vi "raw_to_calibrated-scalar.vi"(5 "tag_name":string, 7 "runtime":variant, 8 "error in (no error)":errorcluster, 11 "value in":dbl) -> (0 "error out":errorcluster, 3 "value out":dbl)   [LabVIEW 2015, in "lv-calibration.lvlib"]
uses:
  lv-calibration.lvlib
  _controls/error.ctl
  <vilib>/gmath/NI_Gmath.lvlib
  <vilib>/Analysis/NI_AALPro.lvlib
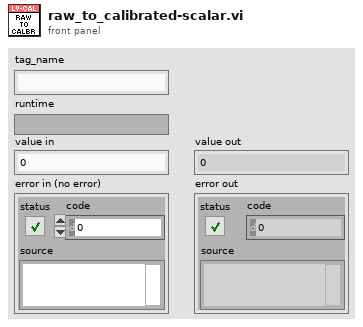
[diagram p1: front panel]
types:
  T1 = typedef "lv-calibration.lvlib/error.ctl" = enum16{"<error>", "unsupported_calibration_type", "tag_name_not_found", "duplicate_tag_names", "formula_empty"}
  T2 = typedef "lv-calibration.lvlib/runtime.ctl" = cluster{"tag_name":string, "type":T3, "offset":dbl, "slope":dbl, "formula":string, "x_points":dbl[], "y_points":dbl[]}
  T3 = typedef "lv-calibration.lvlib/type.ctl" = string
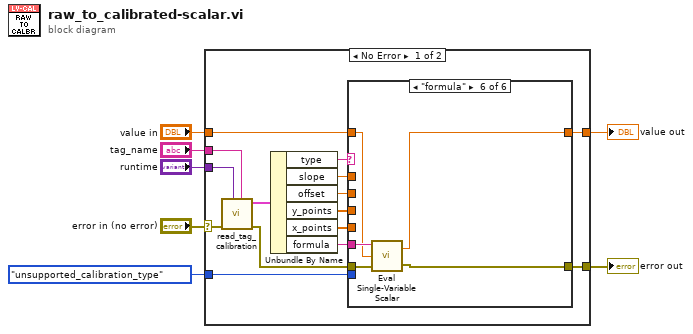
[diagram p0: block diagram]
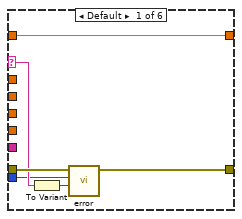
[diagram p2: hidden frame]
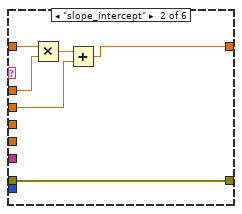
[diagram p3: hidden frame]
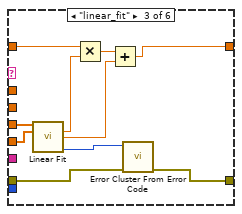
[diagram p4: hidden frame]
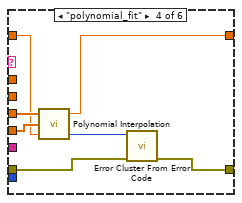
[diagram p5: hidden frame]
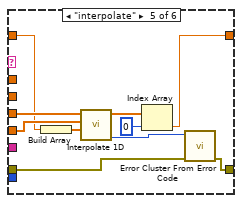
[diagram p6: hidden frame]
diagram:
  n1 = case shown="No Error" "error in (no error)" {
    selector: "error in (no error)" -> [w12 w67]
    tunnel: "value in" -> [w19 _]
    tunnel: [w18 _] -> w6
    tunnel: [w17 w67] -> w5
    tunnel: error."unsupported_calibration_type" ("error") -> [w16 _]
    tunnel: "runtime" -> [w14 _]
    tunnel: "tag_name" -> [w13 _]
    frame No Error {
      n2 = call "read_tag_calibration.vi"("tag_name"=w13, "runtime"=w14, "error in (no error)"=w12) -> ("error out"=w11:errorcluster, "calibration"=w15:T2)  [unwired: 7 in]
      n3 = Unbundle By Name(w15) -> ("type"=w22:T3, "slope"=w21:dbl, "offset"=w20:dbl, "y_points"=w10:dbl[], "x_points"=w9:dbl[], "formula"=w8:string)
      n4 = case shown="\"formula\"" w22 {
        selector: w22 -> [w26 _ _ _ _ _]
        tunnel: w11 -> [w27 w29 w36 w46 w53 w63]
        tunnel: w21 -> [_ w33 _ _ _ _]
        tunnel: w20 -> [_ w32 _ _ _ _]
        tunnel: w19 -> [w28 w34 w40 w49 w59 w65]
        tunnel: [w28 w30 w38 w48 w56 w64] -> w18
        tunnel: [w23 w29 w35 w45 w52 w62] -> w17
        tunnel: w16 -> [w24 _ _ _ _ _]
        tunnel: w10 -> [_ _ w44 w51 w61 _]
        tunnel: w9 -> [_ _ w43 w50 w60 _]
        tunnel: w8 -> [_ _ _ _ _ w66]
        frame Default {
          n5 = To Variant(anything=w26) -> (Variant=w25:variant)
          n6 = call "error.vi"("data"=w25, "error"=w24, "error in (no error)"=w27) -> ("error out"=w23:errorcluster)  [unwired: 8 in]
        }
        frame "slope_intercept" {
          n7 = Multiply(x=w34, y=w33) -> (x*y=w31:dbl)
          n8 = Add(x=w31, y=w32) -> (x+y=w30:dbl)
        }
        frame "linear_fit" {
          n9 = call <vilib>:"Linear Fit.vi"("Y"=w44, "X"=w43) -> ("slope"=w41:dbl, "intercept"=w39:dbl, "error"=w37:i32)  [unwired: 9 in, 2 out]
          n10 = Multiply(x=w40, y=w41) -> (x*y=w42:dbl)
          n11 = Add(x=w42, y=w39) -> (x+y=w38:dbl)
          n12 = call <vilib>:"Error Cluster From Error Code.vi"("error in (no error)"=w36, "error code (0)"=w37) -> ("error out"=w35:errorcluster)  [unwired: 7 in]
        }
        frame "polynomial_fit" {
          n13 = call <vilib>:"Polynomial Interpolation.vi"("x value"=w49, "X"=w50, "Y"=w51) -> ("error"=w47:i32, "interpolation value"=w48:dbl)  [unwired: 1 out]
          n14 = call <vilib>:"Error Cluster From Error Code.vi"("error in (no error)"=w46, "error code (0)"=w47) -> ("error out"=w45:errorcluster)  [unwired: 7 in]
        }
        frame "interpolate" {
          n15 = Build Array(w59) -> (w58:dbl[])
          n16 = call <vilib>:"Interpolate 1D.vi"("xi"=w58, "X"=w60, "Y"=w61) -> ("error"=w54:i32, "yi"=w57:dbl[])  [unwired: 6 in, 1 out]
          n17 = Index Array(array=w57, index=0) -> (element=w56:dbl)
          n18 = call <vilib>:"Error Cluster From Error Code.vi"("error in (no error)"=w53, "error code (0)"=w54) -> ("error out"=w52:errorcluster)  [unwired: 7 in]
        }
        frame "formula" {
          n19 = call <vilib>:"Eval Single-Variable Scalar.vi"("error in (no error)"=w63, "x value"=w65, "formula"=w66) -> ("error out"=w62:errorcluster, "y value"=w64:dbl)
        }
      }
    }
    frame Error {
    }
  }
  "error out" <- w5
  "value out" <- w6
